vi "set_calibration.vi"(6 "timeout (25000ms)":i32=25000, 8 "error in (no error)":errorcluster, 9 "values":dbl[](array[numeric]) format="%#.8g", 10 "calibration":T1[](array[typedef]), 11 "daemon reference in":refnum<k5>) -> (0 "error out":errorcluster, 2 "response":string, 3 "daemon reference out":refnum<k5>, 5 "command out":string="random")   [LabVIEW 2017]
doc: "<b>Command: </b>\"set_calibration\"\n\n<b>Description: </b> Instructs the target to set the specified calibration parameter values.\n\n<b>Parameters: </b> \n\n 1. Parameter Array [max 20]\n 2. Value Array\n____________________________________________\nDIPC 692 Daemon API 10.0.0.1\nSam Tee - Dyson Technology Ltd\nCopyright (c) 2024, Dyson Technology Ltd"
uses:
  typdef/calibration.ctl
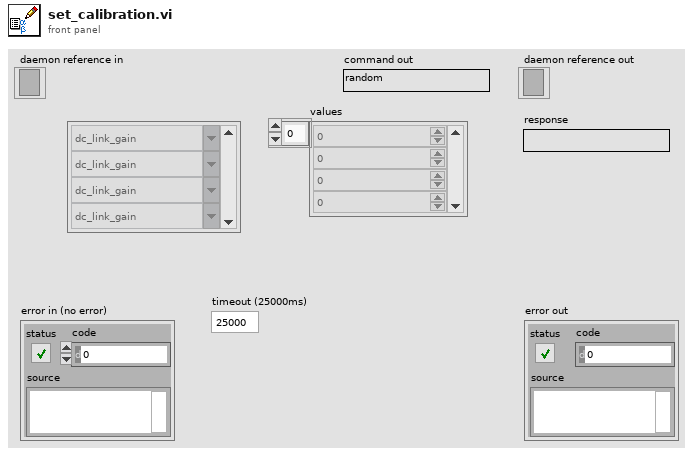
[diagram p1: front panel]
types:
  T1 = typedef "calibration.ctl" = string
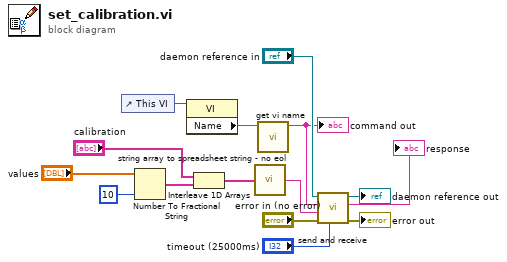
[diagram p0: block diagram]
diagram:
  n1 = control-ref of="This VI"() -> (w10:refnum<vi>)
  n2 = Number To Fractional String(number="values", precision (6)=i16 10) -> (F-format string=w6:string[])  [unwired: 2 in]
  n3 = property class="VI"(reference=w10) -> ("Name"=w9:string)  [unwired: 1 in, 2 out]
  n4 = Interleave 1D Arrays("calibration", w6) -> (w5:T1[])
  n5 = call "string array to spreadsheet string - no eol.vi"("string array"=w5) -> ("spreadsheet string - no eol"=w4:string)
  n6 = call "get vi name.vi"("library.lvlib:name.vi"=w9) -> ("vi name"=w8:string)  [unwired: 10 in]
  "command out" <- w8
  n7 = call "send and receive.vi"("timeout (25000ms)"="timeout (25000ms)", "error in (no error)"="error in (no error)", "data"=w4, "command"=w8, "daemon reference in"="daemon reference in") -> ("error out"=→"error out":errorcluster, "response"=→"response":string, "daemon reference out"=→"daemon reference out":refnum<k5>)  [unwired: 4 in]
